vi "Get Structure Names.vi"(7 "Use Cached Data?":bool, 8 "Error In":errorcluster, 11 "Nest Config":T1) -> (0 "Error Out":errorcluster, 2 "Strcuture Names":string[](array[string]), 3 "Nest Config":T1)   [LabVIEW 2013, in "LVH-Nest.lvlib"]
doc: "Get the names of all structures associated with the Nest account."
uses:
  LVH-Nest.lvlib
  Private/Type Defs/Nest Config.ctl
  <vilib>/httpClient/ClientHandle.ctl
  Private/Type Defs/Session Data.ctl
  <vilib>/httpClient/LabVIEWHTTPClient.lvlib
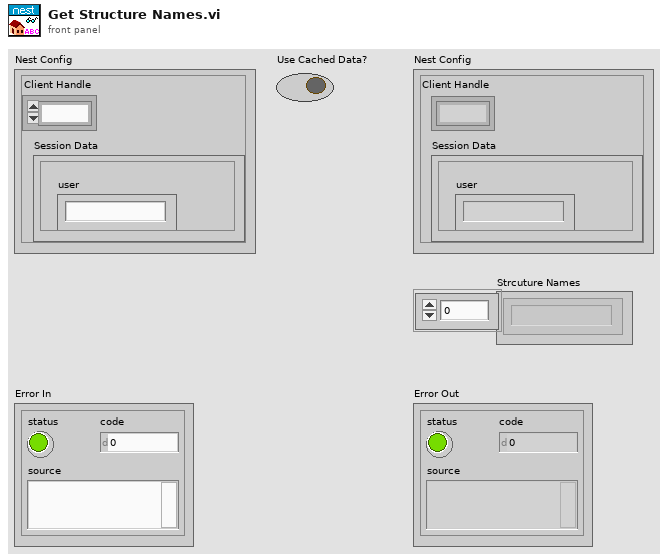
[diagram p1: front panel]
types:
  T1 = typedef "LVH-Nest.lvlib/Nest Config.ctl" = cluster{"Client Handle":T2, "Session Data":T3}
  T2 = typedef "LabVIEWHTTPClient.lvlib/ClientHandle.ctl" = refnum<k1>
  T3 = typedef "LVH-Nest.lvlib/Session Data.ctl" = cluster{"is_superuser":bool, "is_staff":bool, "urls":cluster{"transport_url":string, "rubyapi_url":string, "weather_url":string, "log_upload_url":string, "support_url":string}, "limits":cluster{"thermostats_per_structure":u32, "structures":u32, "thermostats":u32, "smoke_detectors":u32, "smoke_detectors_per_structure":u32}, "access_token":string, "userid":string, "expires_in":string, "email":string, "user":string, "language":string}
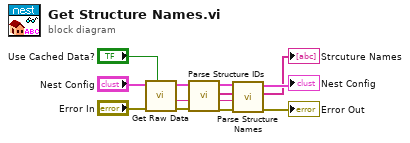
[diagram p0: block diagram]
diagram:
  n1 = call "Get Raw Data.vi"("Use Cached Data?"="Use Cached Data?", "Error In"="Error In", "Nest Config"="Nest Config") -> ("Error Out"=w13:errorcluster, "Data"=w12:string, "Nest Config"=w11:T1)  [unwired: 6 in]
  n2 = call "Parse Structure IDs.vi"("Error In"=w13, "Data"=w12, "Nest Config"=w11) -> ("Error Out"=w7:errorcluster, "Data"=w8:string, "Structure IDs"=w9:string[], "Nest Config"=w10:T1)  [unwired: 5 in]
  n3 = call "Parse Structure Names.vi"("Error In"=w7, "Data"=w8, "Structure IDs"=w9, "Nest Config"=w10) -> ("Error Out"=→"Error Out":errorcluster, "Structure Names"=→"Strcuture Names":string[], "Nest Config"=→"Nest Config":T1)  [unwired: 4 in, 1 out]
